vi "MH_ExtFPGAUserCommand.vi"(8 "error in (no error)":errorcluster, 9 "addr":u32, 10 "write":i32, 11 "devidx":i32) -> (0 "error out":errorcluster, 2 "data":u32, 3 "return type":i32)   [LabVIEW 2019]
uses:
  MH_DllPath_global.vi
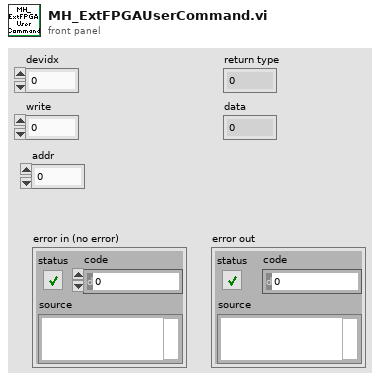
[diagram p1: front panel]
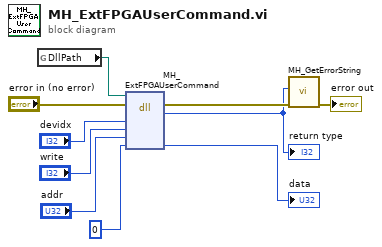
[diagram p0: block diagram]
diagram:
  n1 = global read "MH_DllPath_global.vi" "DllPath"() -> (w9:path)
  n2 = dll-call lib="MHLib64.dll" fn="MH_ExtFPGAUserCommand"(path in=w9, error in="error in (no error)", "devidx"="devidx", "write"="write", "addr"="addr", "data"=u32 0 ("rate")) -> (error out=w7:errorcluster, "return type"=w6:i32, "data"=→"data":u32)  [unwired: 4 in, 1 out]
  "return type" <- w6
  n3 = call "MH_GetErrorString.vi"("error in (no error)"=w7, "code"=w6) -> ("error out"=→"error out":errorcluster)  [unwired: 7 in, 2 out]
